vi "GT_ButIO.vi"(6 "Bule":bool, 7 "doType":i16(ring) items=["MC_ENABLE", "MC_CLEAR", "MC_GPO"], 8 "IO Port":i32, 9 "fifo":i16, 10 "crd":i16, 11 "rtn_In":cluster{"rtn":i16, "Func":string}) -> (1 "fifo out":i16, 2 "crd out":i16, 3 "rtn_Out":cluster{"rtn":i16, "Func":string})   [LabVIEW 2014]
uses:
  VC6/gts.dll
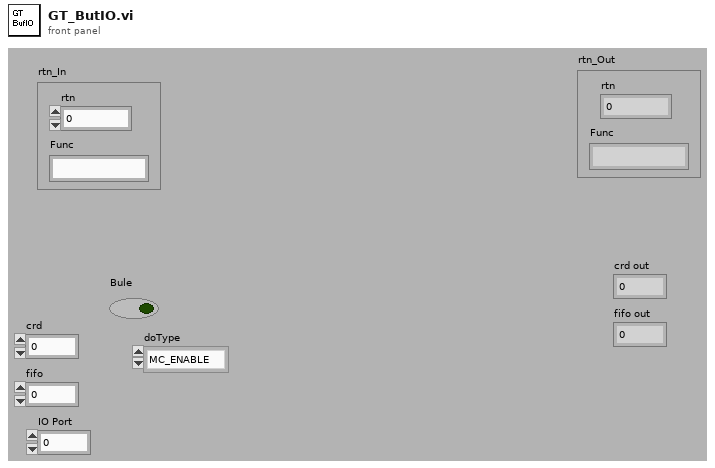
[diagram p1: front panel]
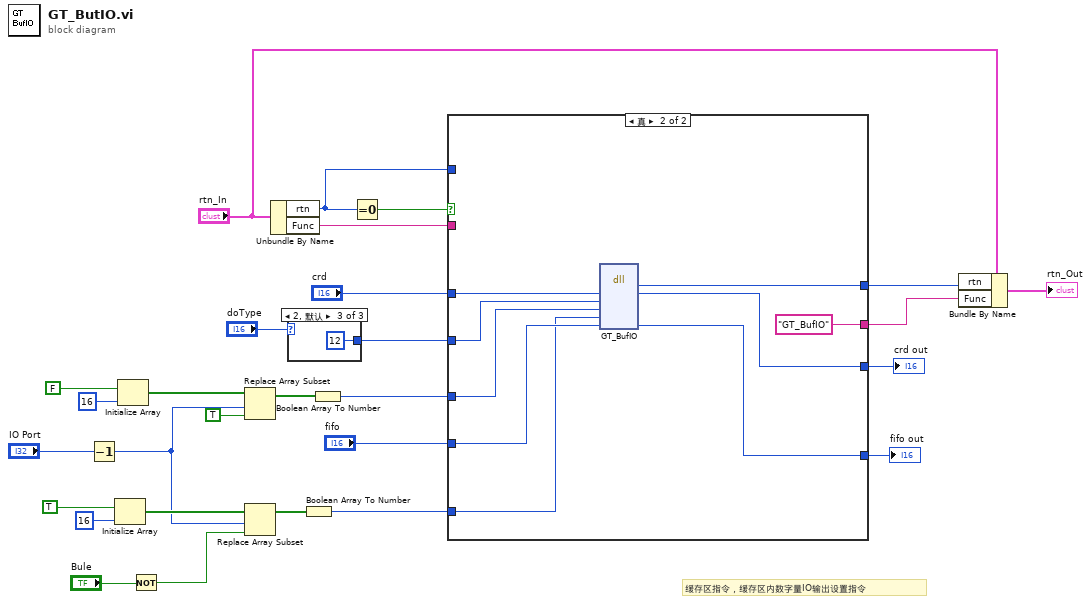
[diagram p0: block diagram]
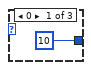
[diagram p2: hidden frame]
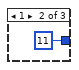
[diagram p3: hidden frame]
diagram:
  # "缓存区指令，缓存区内数字量IO输出设置指令"
  n1 = Decrement(x="IO Port") -> (x-1=w1:i32)
  n2 = Initialize Array(TRUE, 16 ("维数大小")) -> (w9:bool[])
  n3 = Initialize Array(FALSE, 16 ("维数大小")) -> (w13:bool[])
  n4 = Not(x="Bule") -> (.not. x?=w7:bool)
  n5 = Replace Array Subset(array=w13, new element=TRUE, index=w1) -> (w6:bool[])
  n6 = Replace Array Subset(array=w9, new element=w7, index=w1) -> (w4:bool[])
  n7 = Unbundle By Name("rtn_In") -> ("rtn"=w22:i16, "Func"=w23:string)
  n8 = case shown="2, 默认" "doType" {
    tunnel: [i16 10 ("doType") i16 11 ("doType") i16 12 ("doType")] -> w16
    frame 0 {
    }
    frame 1 {
    }
    frame 2, Default {
    }
  }
  n9 = Boolean Array To Number(Boolean array=w4) -> (number=w3:u32)
  n10 = Boolean Array To Number(Boolean array=w6) -> (number=w5:u32)
  n11 = Equal To 0?(x=w22) -> (x = 0?=w28:bool)
  n12 = case shown="真" w28 {
    tunnel: [w34 w44] -> w25
    tunnel: [w35 "GT_BufIO" ("Func")] -> w24
    tunnel: w23 -> [w35 _]
    tunnel: w22 -> [w34 _]
    tunnel: "crd" -> [w33 w42]
    tunnel: [w33 w41] -> w20
    tunnel: "fifo" -> [w32 w40]
    tunnel: [w32 w39] -> w18
    tunnel: w16 -> [_ w38]
    tunnel: w5 -> [_ w37]
    tunnel: w3 -> [_ w36]
    frame False {
    }
    frame True {
      n13 = dll-call lib="PTH2Fabs DNewGTS AC-800LWin7版源程序-20170926gts85VC6gts.dll" fn="GT_BufIO"("crd"=w42, "doType"=w38, "doMask"=w37, "doValue"=w36, "fifo"=w40) -> ("rtn"=w44:i16, "crd"=w41:i16, "fifo"=w39:i16)  [unwired: 6 in, 2 out]
    }
  }
  "crd out" <- w20
  "fifo out" <- w18
  n14 = Bundle By Name(cluster="rtn_In", "rtn"=w25, "Func"=w24) -> (→"rtn_Out":cluster{"rtn":i16, "Func":string})
